vi "Begin.vi"() -> ()   [LabVIEW 2011]
doc: "Called before other user functions, this VI is expected to open initial I/O refnums, load in file data, and do all program initialization. Notice that the <B>error out</B> terminal is simply used for data flow. Wiring it to other structures or subVIs ensures that this VI runs first."
uses:
  <vilib>/Rock Robotics/SystemInterfaces/DIO/FPGA_DIOPWMChannel.ctl
  <vilib>/Rock Robotics/WPI/Joystick/WPI_JoystickDeviceEnum.ctl
  <vilib>/Rock Robotics/SystemInterfaces/AI/FPGA_AIChannel.ctl
  <vilib>/Rock Robotics/SystemInterfaces/DIO/FPGA_DIORelayChannel.ctl
  <vilib>/Rock Robotics/SystemInterfaces/DIO/FPGA_DIOChannel.ctl
  <vilib>/Rock Robotics/SystemInterfaces/AI/FPGA_AIGyroChannel.ctl
  <vilib>/Rock Robotics/WPI/Relay/WPI_RelayDirection.ctl
  <vilib>/Rock Robotics/WPI/Encoder/WPI_EncoderType.ctl
  <vilib>/Rock Robotics/WPI/DriverStation/DriverStationLCD/WPI_DriverStationLCDLCDLine.ctl
  <vilib>/Rock Robotics/WPI/MotorControl/WPI_MotorControlOpen Victor.vi
  <vilib>/Rock Robotics/WPI/MotorControl/WPI_MotorControlOpen Jaguar.vi
  GLOBALShooter.vi
  <vilib>/Rock Robotics/WPI/Counter/WPI_CounterDigitalInputToDigitalSource.vi
  GLOBALHarvester.vi
  <vilib>/Rock Robotics/WPI/RobotDrive/WPI_RobotDriveOpen2MotorWithJaguar.vi
  GLOBALVision.vi
  GLOBALMain.vi
panel:
  in  "Default Shooter in Feet 2":i32=13
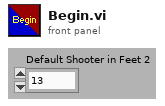
[diagram p1: front panel]
types:
  T1 = typedef "FPGA_DIOPWMChannel.ctl" = enum8{"PWM 1", "PWM 2", "PWM 3", "PWM 4", "PWM 5", "PWM 6", "PWM 7", "PWM 8", "PWM 9", "PWM 10", "Invalid"}
  T2 = typedef "WPI_DriverStationLCDLCDLine.ctl" = enum16{"Main - Line 1", "User - Line 2", "User - Line 3", "User - Line 4", "User - Line 5", "User - Line 6"}
  T3 = typedef "WPI_EncoderType.ctl" = enum16{"1x", "2x", "4x"}
  T4 = typedef "FPGA_DIOChannel.ctl" = enum8{"DIO 1", "DIO 2", "DIO 3", "DIO 4", "DIO 5", "DIO 6", "DIO 7", "DIO 8", "DIO 9", "DIO 10", "DIO 11", "DIO 12", "DIO 13", "DIO 14", "Invalid"}
  T5 = typedef "FPGA_DIORelayChannel.ctl" = enum8{"Relay 1", "Relay 2", "Relay 3", "Relay 4", "Relay 5", "Relay 6", "Relay 7", "Relay 8", "Invalid"}
  T6 = typedef "WPI_RelayDirection.ctl" = enum16{"Both directions", "Forward only", "Reverse only"}
  T7 = typedef "FPGA_AIGyroChannel.ctl" = enum8{"AI 1", "AI 2", "Invalid"}
  T8 = typedef "FPGA_AIChannel.ctl" = enum8{"AI 1", "AI 2", "AI 3", "AI 4", "AI 5", "AI 6", "AI 7", "AI 8", "Invalid"}
  T9 = typedef "WPI_JoystickDeviceEnum.ctl" = enum16{"USB 1", "USB 2", "USB 3", "USB 4", "Kinect 1", "Kinect 2"}
  T10 = typedef "WPI_MotorControlDeviceRef.ctl" = cluster{"DeviceStatus":errorcluster, "Type":enum16{"PWM", "CAN"}, "PWM":cluster{"Digital Module":T11, "PWM Channel":T1, "DeadBand":T12}, "CAN":cluster{"Device Number":u8, "Control Mode":T13, "Semaphore":T14, "Max Vout":dbl}, "Invert":bool, "TransformRef":T15, "InvTransformRef":T15}
  T11 = typedef "FPGA_TypedefDigitalModule.ctl" = enum16{"Digital Module 1", "Digital Module 2"}
  T12 = typedef "WPI_PWMDeadband.ctl" = cluster{"Name":string, "maxPositivePwm":i32, "minPositivePwm":i32, "centerPwm":i32, "maxNegativePwm":i32, "minNegativePwm":i32, "angularRange":u16}
  T13 = typedef "WPI_CANJaguar_ControlMode.ctl" = enum8{"Percent VBus", "Current", "Speed", "Position", "Voltage"}
  T14 = typedef "Semaphore RefNum" = refnum<k1>
  T15 = typedef "WPI_PWMTransform_ConPane.ctl" = refnum<vi>
  T16 = typedef "WPI_RobotDriveDevRef.ctl" = cluster{"DevStatus":errorcluster, "Motors[]":T10[], "Square Inputs":bool, "Max Output":dbl, "Isochronous":bool}
  T17 = typedef "WPI_AnalogChannelDevRef.ctl" = cluster{"DevStatus":errorcluster, "Analog Module":T18, "Analog Channel":T8}
  T18 = typedef "FPGA_TypedefAnalogModule.ctl" = enum16{"Analog Module 1", "Analog Module 2"}
  T19 = typedef "WPI_CameraImageSize.ctl" = enum16{"640x480", "320x240", "160x120"}
  T20 = typedef "WPI_CameraWhite Balance Values.ctl" = enum16{"Auto", "Fixed indoor", "Fixed outdoor 1", "Fixed outdoor 2", "Fixed fluorescent 1", "Fixed fluorescent 2", "Hold current"}
  T21 = typedef "WPI_CameraExposure Values.ctl" = enum16{"Auto", "Flicker-free 50 Hz", "Flicker-free 60 Hz", "Hold current"}
  T22 = cluster{"fps":i32, "compression":i32, "Image Size":T19, "Camera Resolultion":cluster{i32, i32}[], "White Balance":T20, "Exposure":T21, "Brightness":dbl, "Enable Color":bool, "Camera Address":string}
  T23 = typedef "WPI_ServoDeviceRef.ctl" = cluster{"DeviceStatus":errorcluster, "Digital Module":T11, "PWM Channel":T1, "DeadBand":T12}
  T24 = typedef "WPI_RelayDevRef.ctl" = cluster{"DevStatus":errorcluster, "Relay Channel":T5, "Digital Module":T11, "Relay Direction":T6}
  T25 = typedef "WPI_JoystickDevRef.ctl" = cluster{"Device":T9}
  T26 = typedef "WPI_DigitalInputDevRef.ctl" = cluster{"DevStatus":errorcluster, "DIO Channel":T4, "Digital Module":T11}
  T27 = typedef "FPGA_CounterEncoderSourceConvertionLVSourceType.ctl" = cluster{"DevStatus":errorcluster, "AnalogTriggerMode?":bool, "DigitalMode":cluster{"Digital Module":T11, "DIO Channel":T28}, "AnalogTriggerMode":cluster{"AnalogTriggerIndex":T29, "OutputType":T30}}
  T28 = typedef "FPGA_DIODigitalSourceChannel.ctl" = enum8{"DIO 1", "DIO 2", "DIO 3", "DIO 4", "DIO 5", "DIO 6", "DIO 7", "DIO 8", "DIO 9", "DIO 10", "DIO 11", "DIO 12", "DIO 13", "DIO 14", "Disabled"}
  T29 = typedef "FPGA_AnalogTriggerIndex.ctl" = enum8{"Trig 0", "Trig 1", "Trig 2", "Trig 3", "Trig 4", "Trig 5", "Trig 6", "Trig 7", "Invalid"}
  T30 = typedef "FPGA_AnalogTriggerOutType.ctl" = enum16{"InWindow", "TriggerState", "Rising", "Falling"}
  T31 = typedef "WPI_GyroDevRef.ctl" = cluster{"DevStatus":errorcluster, "Analog Module":T18, "Analog Channel":T8, "Offset":dbl, "Gain (VoltsPerDegree/Second)":dbl}
  T32 = typedef "WPI_EncoderDevRef.ctl" = cluster{"DevStatus":errorcluster, "EncoderIndex":T33, "CounterIndex":T34, "DistancePerCount":dbl, "Decoding Type":T3}
  T33 = typedef "FPGA_EncoderIdx.ctl" = enum8{"Enc 0", "Enc 1", "Enc 2", "Enc 3", "Invalid"}
  T34 = typedef "FPGA_CounterCtrSystemIndex.ctl" = enum8{"Ctr 0", "Ctr 1", "Ctr 2", "Ctr 3", "Ctr 4", "Ctr 5", "Ctr 6", "Ctr 7", "Invalid"}
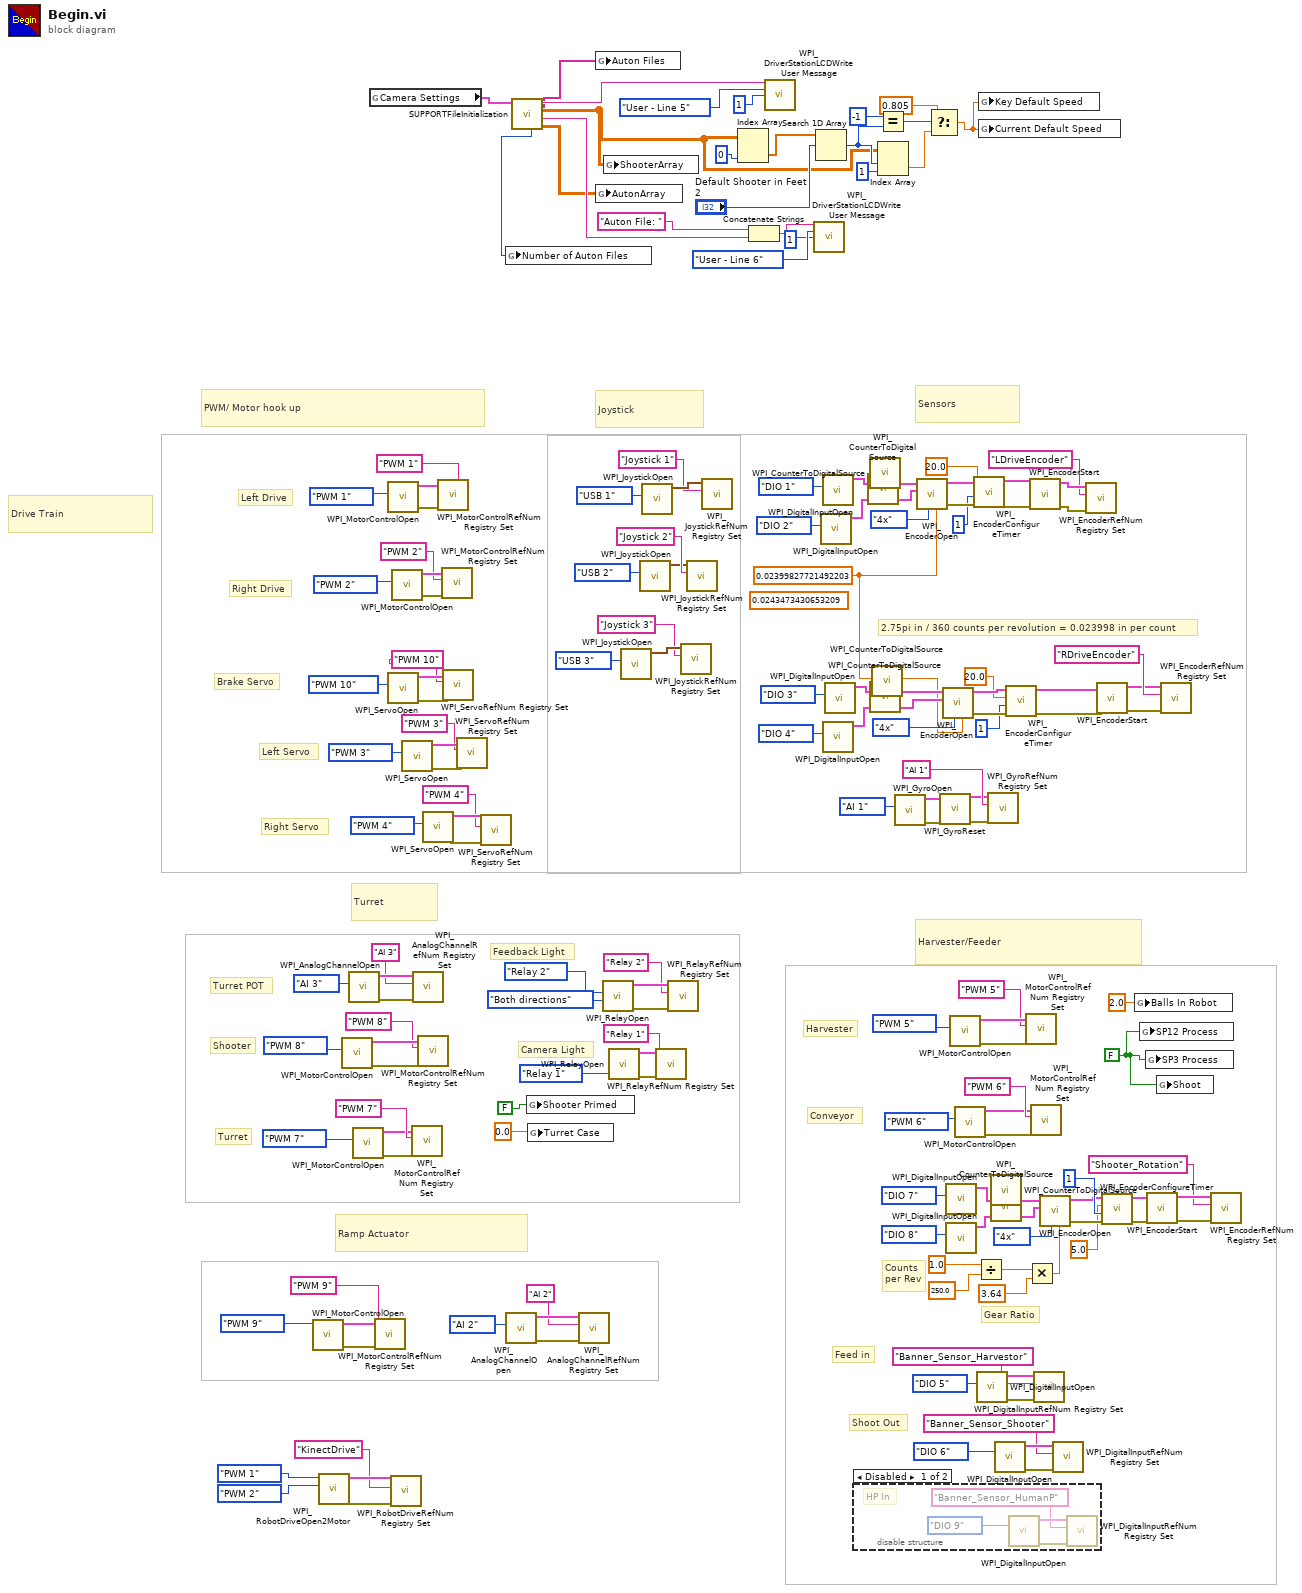
[diagram p0: block diagram]
diagram:
  w29 = FALSE ("Ball S12 Process")
  (unwired) 0.0243473430653209 ("DistancePerCount")
  w58 = 0.02399827721492203 ("DistancePerCount")
  # "Feedback Light"
  # "Brake Servo"
  # "Right Drive"
  # "Left Drive"
  # "Counts\nper Rev"
  # "Gear Ratio"
  # "2.75pi in / 360 counts per revolution = 0.023998 in per count"
  # "Shoot Out"
  # "Feed in"
  # "Harvester"
  # "Conveyor"
  # "Shooter"
  # "Camera Light"
  # "Turret POT"
  # "Turret"
  # "Right Servo"
  # "Left Servo"
  # "Harvester/Feeder"
  # "Turret"
  # "Ramp Actuator"
  # "Drive Train"
  # "Sensors"
  # "Joystick"
  # "PWM/ Motor hook up"
  n1 = call-poly <vilib>:"WPI_MotorControlOpen.vi"("PWM Channel"=FPGA_DIOPWMChannel."PWM 9") -> ("error out"=w128:errorcluster, "MotorControlDeviceRef"=w129:T10)  [unwired: 9 in]
  n2 = call-poly <vilib>:"WPI_RobotDriveOpen2Motor.vi"("Right Motor"=FPGA_DIOPWMChannel."PWM 2", "Left Motor"=FPGA_DIOPWMChannel."PWM 1") -> ("error out"=w4:errorcluster, "RobotDriveDevRef"=w5:T16)  [unwired: 8 in]
  n3 = call-poly <vilib>:"WPI_MotorControlOpen.vi"("PWM Channel"=FPGA_DIOPWMChannel."PWM 8") -> ("error out"=w118:errorcluster, "MotorControlDeviceRef"=w120:T10)  [unwired: 9 in]
  n4 = call <vilib>:"WPI_AnalogChannelOpen.vi"("Analog Channel"=FPGA_AIChannel."AI 3") -> ("error out"=w136:errorcluster, "AIDeviceRef"=w137:T17)  [unwired: 9 in]
  n5 = call-poly <vilib>:"WPI_MotorControlOpen.vi"("PWM Channel"=FPGA_DIOPWMChannel."PWM 7") -> ("error out"=w141:errorcluster, "MotorControlDeviceRef"=w139:T10)  [unwired: 9 in]
  n6 = global read "GLOBALVision.vi" "Camera Settings"() -> (w28:T22)
  n7 = call <vilib>:"WPI_MotorControlRefNum Registry Set.vi"("error in (no error)"=w128, "refnum name"="PWM 9", "MotorControlDevRef"=w129) -> ()  [unwired: 7 in, 2 out]
  n8 = call-poly <vilib>:"WPI_MotorControlOpen.vi"("PWM Channel"=FPGA_DIOPWMChannel."PWM 1") -> ("error out"=w147:errorcluster, "MotorControlDeviceRef"=w149:T10)  [unwired: 9 in]
  n9 = call <vilib>:"WPI_ServoOpen.vi"("PWM Channel"=FPGA_DIOPWMChannel."PWM 10") -> ("error out"=w34:errorcluster, "ServoDeviceRef"=w36:T23)  [unwired: 9 in]
  n10 = call <vilib>:"WPI_RobotDriveRefNum Registry Set.vi"("error in (no error)"=w4, "refnum name"="KinectDrive", "RobotDriveDevRef"=w5) -> ()  [unwired: 7 in, 2 out]
  n11 = call-poly <vilib>:"WPI_MotorControlOpen.vi"("PWM Channel"=FPGA_DIOPWMChannel."PWM 2") -> ("error out"=w145:errorcluster, "MotorControlDeviceRef"=w143:T10)  [unwired: 9 in]
  n12 = call <vilib>:"WPI_ServoOpen.vi"("PWM Channel"=FPGA_DIOPWMChannel."PWM 3") -> ("error out"=w160:errorcluster, "ServoDeviceRef"=w165:T23)  [unwired: 9 in]
  n13 = call <vilib>:"WPI_MotorControlRefNum Registry Set.vi"("error in (no error)"=w141, "refnum name"="PWM 7", "MotorControlDevRef"=w139) -> ()  [unwired: 7 in, 2 out]
  n14 = call <vilib>:"WPI_AnalogChannelRefNum Registry Set.vi"("error in (no error)"=w136, "refnum name"="AI 3", "AIDeviceRef"=w137) -> ()  [unwired: 7 in, 2 out]
  n15 = call <vilib>:"WPI_MotorControlRefNum Registry Set.vi"("error in (no error)"=w118, "refnum name"="PWM 8", "MotorControlDevRef"=w120) -> ()  [unwired: 7 in, 2 out]
  n16 = call <vilib>:"WPI_ServoOpen.vi"("PWM Channel"=FPGA_DIOPWMChannel."PWM 4") -> ("error out"=w159:errorcluster, "ServoDeviceRef"=w163:T23)  [unwired: 9 in]
  n17 = call <vilib>:"WPI_MotorControlRefNum Registry Set.vi"("error in (no error)"=w147, "refnum name"="PWM 1", "MotorControlDevRef"=w149) -> ()  [unwired: 7 in, 2 out]
  n18 = call <vilib>:"WPI_MotorControlRefNum Registry Set.vi"("error in (no error)"=w145, "refnum name"="PWM 2", "MotorControlDevRef"=w143) -> ()  [unwired: 7 in, 2 out]
  n19 = call <vilib>:"WPI_ServoRefNum Registry Set.vi"("error in (no error)"=w34, "refnum name"="PWM 10", "ServoDeviceRef"=w36) -> ()  [unwired: 7 in, 2 out]
  n20 = call <vilib>:"WPI_ServoRefNum Registry Set.vi"("error in (no error)"=w160, "refnum name"="PWM 3", "ServoDeviceRef"=w165) -> ()  [unwired: 7 in, 2 out]
  n21 = call <vilib>:"WPI_ServoRefNum Registry Set.vi"("error in (no error)"=w159, "refnum name"="PWM 4", "ServoDeviceRef"=w163) -> ()  [unwired: 7 in, 2 out]
  n22 = call <vilib>:"WPI_AnalogChannelOpen.vi"("Analog Channel"=FPGA_AIChannel."AI 2") -> ("error out"=w132:errorcluster, "AIDeviceRef"=w133:T17)  [unwired: 9 in]
  n23 = call "SUPPORTFileInitialization.vi"("Camera Info"=w28) -> ("AutonArray"=w8:dbl[][], "Current Auton File"=w9:string, "ShooterArray"=w15:dbl[][], "ShooterFile"=w25:string, "Number of Auton Files"=w7:i64, "Auton Files"=w6:string[])  [unwired: 5 in]
  n24 = global write "GLOBALMain.vi" "Number of Auton Files"(w7) -> ()
  n25 = global write "GLOBALShooter.vi" "Shooter Primed"(FALSE ("Ball S3 Process")) -> ()
  n26 = global write "GLOBALShooter.vi" "Turret Case"(0.0 ("Return To Home Case")) -> ()
  n27 = call <vilib>:"WPI_AnalogChannelRefNum Registry Set.vi"("error in (no error)"=w132, "refnum name"="AI 2", "AIDeviceRef"=w133) -> ()  [unwired: 7 in, 2 out]
  n28 = global write "GLOBALMain.vi" "Auton Files"(w6) -> ()
  n29 = global write "GLOBALMain.vi" "AutonArray"(w8) -> ()
  n30 = call <vilib>:"WPI_RelayOpen.vi"("Relay Direction"=WPI_RelayDirection."Both directions", "Relay Channel"=FPGA_DIORelayChannel."Relay 2") -> ("error out"=w94:errorcluster, "RelayDevRef"=w95:T24)  [unwired: 8 in]
  n31 = global write "GLOBALShooter.vi" "ShooterArray"(w15) -> ()
  n32 = call <vilib>:"WPI_RelayOpen.vi"("Relay Channel"=FPGA_DIORelayChannel."Relay 1") -> ("error out"=w125:errorcluster, "RelayDevRef"=w124:T24)  [unwired: 9 in]
  n33 = call <vilib>:"WPI_JoystickOpen.vi"("JoystickDevice"=WPI_JoystickDeviceEnum."USB 3") -> ("JoystickDevRef"=w152:T25)  [unwired: 10 in]
  n34 = call <vilib>:"WPI_JoystickOpen.vi"("JoystickDevice"=WPI_JoystickDeviceEnum."USB 2") -> ("JoystickDevRef"=w155:T25)  [unwired: 10 in]
  n35 = call <vilib>:"WPI_JoystickOpen.vi"("JoystickDevice"=WPI_JoystickDeviceEnum."USB 1") -> ("JoystickDevRef"=w158:T25)  [unwired: 10 in]
  n36 = call <vilib>:"WPI_RelayRefNum Registry Set.vi"("error in (no error)"=w125, "refnum name"="Relay 1", "RelayDevRef"=w124) -> ()  [unwired: 7 in, 2 out]
  n37 = call <vilib>:"WPI_RelayRefNum Registry Set.vi"("error in (no error)"=w94, "refnum name"="Relay 2", "RelayDevRef"=w95) -> ()  [unwired: 7 in, 2 out]
  n38 = call <vilib>:"WPI_JoystickRefNum Registry Set.vi"("refnum name"="Joystick 3", "JoystickDevRef"=w152) -> ()  [unwired: 8 in, 2 out]
  n39 = call <vilib>:"WPI_JoystickRefNum Registry Set.vi"("refnum name"="Joystick 2", "JoystickDevRef"=w155) -> ()  [unwired: 8 in, 2 out]
  n40 = call <vilib>:"WPI_JoystickRefNum Registry Set.vi"("refnum name"="Joystick 1", "JoystickDevRef"=w158) -> ()  [unwired: 8 in, 2 out]
  n41 = Index Array(array=w15, index (col)=0 ("disabled index (col)")) -> (element=w18:dbl[])  [unwired: 1 in]
  n42 = Concatenate Strings("Auton File: ", w9) -> (w13:string)
  n43 = call <vilib>:"WPI_DriverStationLCDWrite User Message.vi"("line text"=w25, "line"=WPI_DriverStationLCDLCDLine."User - Line 5", "starting column"=i8 1) -> ()  [unwired: 2 in, 11 out]
  n44 = call <vilib>:"WPI_DriverStationLCDWrite User Message.vi"("line text"=w13, "line"=WPI_DriverStationLCDLCDLine."User - Line 6", "starting column"=i8 1) -> ()  [unwired: 2 in, 11 out]
  n45 = Search 1D Array(1D array=w18, element="Default Shooter in Feet 2") -> (index of element=w21:i32)  [unwired: 1 in]
  n46 = call <vilib>:"WPI_DigitalInputOpen.vi"("DIO Channel"=FPGA_DIOChannel."DIO 2") -> ("DigitalInputDevRef"=w86:T26)  [unwired: 9 in, 1 out]
  n47 = call <vilib>:"WPI_DigitalInputOpen.vi"("DIO Channel"=FPGA_DIOChannel."DIO 1") -> ("DigitalInputDevRef"=w83:T26)  [unwired: 9 in, 1 out]
  n48 = call <vilib>:"WPI_DigitalInputOpen.vi"("DIO Channel"=FPGA_DIOChannel."DIO 4") -> ("DigitalInputDevRef"=w77:T26)  [unwired: 9 in, 1 out]
  n49 = call <vilib>:"WPI_DigitalInputOpen.vi"("DIO Channel"=FPGA_DIOChannel."DIO 3") -> ("DigitalInputDevRef"=w80:T26)  [unwired: 9 in, 1 out]
  n50 = disable-structure shown="Disabled" {
    frame Disabled {
      # "HP In"
      n51 = call <vilib>:"WPI_DigitalInputOpen.vi"("DIO Channel"=FPGA_DIOChannel."DIO 9") -> ("error out"=w169:errorcluster, "DigitalInputDevRef"=w168:T26)  [unwired: 9 in]
      n52 = call <vilib>:"WPI_DigitalInputRefNum Registry Set.vi"("error in (no error)"=w169, "refnum name"="Banner_Sensor_HumanP", "DigitalInputDevRef"=w168) -> ()  [unwired: 7 in, 2 out]
    }
    frame Enabled {
    }
  }
  n53 = call-poly <vilib>:"WPI_CounterToDigitalSource.vi"("DigitalInputDevRef"=w86) -> ("Digital Source"=w87:T27)  [unwired: 6 in]
  n54 = call-poly <vilib>:"WPI_CounterToDigitalSource.vi"("DigitalInputDevRef"=w83) -> ("Digital Source"=w82:T27)  [unwired: 6 in]
  n55 = call-poly <vilib>:"WPI_CounterToDigitalSource.vi"("DigitalInputDevRef"=w77) -> ("Digital Source"=w76:T27)  [unwired: 6 in]
  n56 = call-poly <vilib>:"WPI_CounterToDigitalSource.vi"("DigitalInputDevRef"=w80) -> ("Digital Source"=w81:T27)  [unwired: 6 in]
  n57 = Equal?(x=-1, y=w21) -> (x = y?=w23:bool)
  n58 = Index Array(array=w15, index (row)=w21, index (col)=1) -> (element=w16:dbl)
  n59 = call <vilib>:"WPI_GyroOpen.vi"("Analog Channel"=FPGA_AIGyroChannel."AI 1") -> ("error out"=w98:errorcluster, "GyroDevRef"=w99:T31)  [unwired: 8 in, 1 out]
  n60 = call <vilib>:"WPI_EncoderOpen.vi"("DistancePerCount"=w58, "Decoding Type"=WPI_EncoderType."4x", "BSource"=w87, "ASource"=w82) -> ("error out"=w62:errorcluster, "EncoderDevRef"=w65:T32)  [unwired: 6 in]
  n61 = Select(t=0.805, s=w23, f=w16) -> (s? t:f=w14:dbl)
  n62 = call <vilib>:"WPI_GyroReset.vi"("error in (no error)"=w98, "GyroDevRef"=w99) -> ("error out"=w97:errorcluster, "GyroDevRef"=w96:T31)  [unwired: 8 in]
  n63 = call <vilib>:"WPI_EncoderOpen.vi"("DistancePerCount"=w58, "Decoding Type"=WPI_EncoderType."4x", "BSource"=w76, "ASource"=w81) -> ("error out"=w73:errorcluster, "EncoderDevRef"=w72:T32)  [unwired: 6 in]
  n64 = call <vilib>:"WPI_DigitalInputOpen.vi"("DIO Channel"=FPGA_DIOChannel."DIO 7") -> ("DigitalInputDevRef"=w42:T26)  [unwired: 9 in, 1 out]
  n65 = call <vilib>:"WPI_DigitalInputOpen.vi"("DIO Channel"=FPGA_DIOChannel."DIO 8") -> ("DigitalInputDevRef"=w45:T26)  [unwired: 9 in, 1 out]
  n66 = call-poly <vilib>:"WPI_MotorControlOpen.vi"("PWM Channel"=FPGA_DIOPWMChannel."PWM 5") -> ("error out"=w114:errorcluster, "MotorControlDeviceRef"=w116:T10)  [unwired: 9 in]
  n67 = call-poly <vilib>:"WPI_MotorControlOpen.vi"("PWM Channel"=FPGA_DIOPWMChannel."PWM 6") -> ("error out"=w113:errorcluster, "MotorControlDeviceRef"=w111:T10)  [unwired: 9 in]
  n68 = call <vilib>:"WPI_EncoderConfigureTimer.vi"("error in (no error)"=w62, "Number Samples to Average"=u8 1, "Minimum Rate"=20.0, "EncoderDevRef"=w65) -> ("error out"=w63:errorcluster, "EncoderDevRef"=w64:T32)  [unwired: 6 in]
  n69 = Divide(x=1.0, y=250.0) -> (x/y=w39:dbl)
  n70 = call <vilib>:"WPI_DigitalInputOpen.vi"("DIO Channel"=FPGA_DIOChannel."DIO 5") -> ("error out"=w107:errorcluster, "DigitalInputDevRef"=w106:T26)  [unwired: 9 in]
  n71 = global write "GLOBALShooter.vi" "Key Default Speed"(w14) -> ()
  n72 = global write "GLOBALShooter.vi" "Current Default Speed"(w14) -> ()
  n73 = call <vilib>:"WPI_GyroRefNum Registry Set.vi"("error in (no error)"=w97, "refnum name"="AI 1", "GyroDevRef"=w96) -> ()  [unwired: 7 in, 2 out]
  n74 = call-poly <vilib>:"WPI_CounterToDigitalSource.vi"("DigitalInputDevRef"=w42) -> ("Digital Source"=w41:T27)  [unwired: 6 in]
  n75 = call-poly <vilib>:"WPI_CounterToDigitalSource.vi"("DigitalInputDevRef"=w45) -> ("Digital Source"=w46:T27)  [unwired: 6 in]
  n76 = call <vilib>:"WPI_DigitalInputOpen.vi"("DIO Channel"=FPGA_DIOChannel."DIO 6") -> ("error out"=w104:errorcluster, "DigitalInputDevRef"=w103:T26)  [unwired: 9 in]
  n77 = call <vilib>:"WPI_EncoderConfigureTimer.vi"("error in (no error)"=w73, "Number Samples to Average"=u8 1, "Minimum Rate"=20.0, "EncoderDevRef"=w72) -> ("error out"=w69:errorcluster, "EncoderDevRef"=w70:T32)  [unwired: 6 in]
  n78 = call <vilib>:"WPI_MotorControlRefNum Registry Set.vi"("error in (no error)"=w114, "refnum name"="PWM 5", "MotorControlDevRef"=w116) -> ()  [unwired: 7 in, 2 out]
  n79 = Multiply(x=w39, y=3.64) -> (x*y=w37:dbl)
  n80 = call <vilib>:"WPI_EncoderStart.vi"("error in (no error)"=w63, "EncoderDevRef"=w64) -> ("error out"=w90:errorcluster, "EncoderDevRef"=w89:T32)  [unwired: 8 in]
  n81 = call <vilib>:"WPI_MotorControlRefNum Registry Set.vi"("error in (no error)"=w113, "refnum name"="PWM 6", "MotorControlDevRef"=w111) -> ()  [unwired: 7 in, 2 out]
  n82 = call <vilib>:"WPI_DigitalInputRefNum Registry Set.vi"("error in (no error)"=w107, "refnum name"="Banner_Sensor_Harvestor", "DigitalInputDevRef"=w106) -> ()  [unwired: 7 in, 2 out]
  n83 = call <vilib>:"WPI_EncoderOpen.vi"("DistancePerCount"=w37, "Decoding Type"=WPI_EncoderType."4x", "BSource"=w46, "ASource"=w41) -> ("error out"=w49:errorcluster, "EncoderDevRef"=w50:T32)  [unwired: 6 in]
  n84 = call <vilib>:"WPI_DigitalInputRefNum Registry Set.vi"("error in (no error)"=w104, "refnum name"="Banner_Sensor_Shooter", "DigitalInputDevRef"=w103) -> ()  [unwired: 7 in, 2 out]
  n85 = call <vilib>:"WPI_EncoderRefNum Registry Set.vi"("error in (no error)"=w90, "refnum name"="LDriveEncoder", "EncoderDevRef"=w89) -> ()  [unwired: 7 in, 2 out]
  n86 = call <vilib>:"WPI_EncoderStart.vi"("error in (no error)"=w69, "EncoderDevRef"=w70) -> ("error out"=w67:errorcluster, "EncoderDevRef"=w68:T32)  [unwired: 8 in]
  n87 = call <vilib>:"WPI_EncoderConfigureTimer.vi"("error in (no error)"=w49, "Number Samples to Average"=u8 1, "Minimum Rate"=5.0, "EncoderDevRef"=w50) -> ("error out"=w53:errorcluster, "EncoderDevRef"=w52:T32)  [unwired: 6 in]
  n88 = global write "GLOBALHarvester.vi" "Balls In Robot"(2.0 ("Balls In Robot")) -> ()
  n89 = global write "GLOBALHarvester.vi" "SP12 Process"(w29) -> ()
  n90 = global write "GLOBALHarvester.vi" "SP3 Process"(w29) -> ()
  n91 = call <vilib>:"WPI_EncoderStart.vi"("error in (no error)"=w53, "EncoderDevRef"=w52) -> ("error out"=w55:errorcluster, "EncoderDevRef"=w54:T32)  [unwired: 8 in]
  n92 = global write "GLOBALHarvester.vi" "Shoot"(w29) -> ()
  n93 = call <vilib>:"WPI_EncoderRefNum Registry Set.vi"("error in (no error)"=w67, "refnum name"="RDriveEncoder", "EncoderDevRef"=w68) -> ()  [unwired: 7 in, 2 out]
  n94 = call <vilib>:"WPI_EncoderRefNum Registry Set.vi"("error in (no error)"=w55, "refnum name"="Shooter_Rotation", "EncoderDevRef"=w54) -> ()  [unwired: 7 in, 2 out]
